vi "Acknowledge Message.vi"(6 "Acknowledge Data":T1, 8 "error in":errorcluster, 9 "Module Action":string, 11 "Module Data In":refnum<class "Rename.lvclass">) -> (0 "error out":errorcluster, 3 "Module Data Out":refnum<class "Rename.lvclass">)   [LabVIEW 2015, in "Generic Module Library.lvlib" / "Template G_Module.lvlib"]
uses:
  Template G_Module.lvlib
  Private Controls/Module Message Cluster Components/Acknowledge Data Cluster.ctl
  Module Class/Rename.lvclass
  Private Controls/Module Message Cluster Components/Ack Payload.ctl
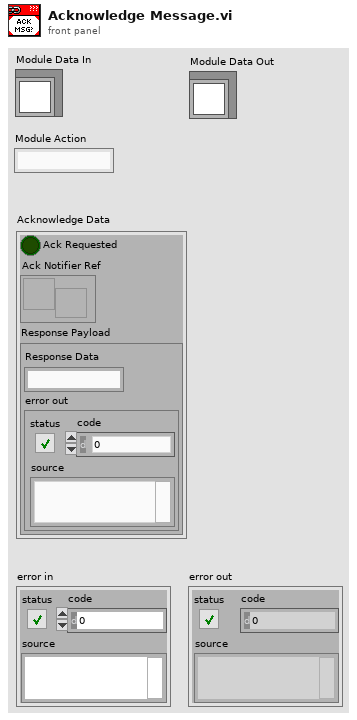
[diagram p1: front panel]
types:
  T1 = typedef "Generic Module Library.lvlib/Template G_Module.lvlib/Acknowledge Data Cluster.ctl" = cluster{"Ack Requested":bool, "Ack Notifier Ref":refnum<notifier>, "Response Payload":T2}
  T2 = typedef "Generic Module Library.lvlib/Template G_Module.lvlib/Ack Payload.ctl" = cluster{"Response Data":string, "error out":errorcluster}
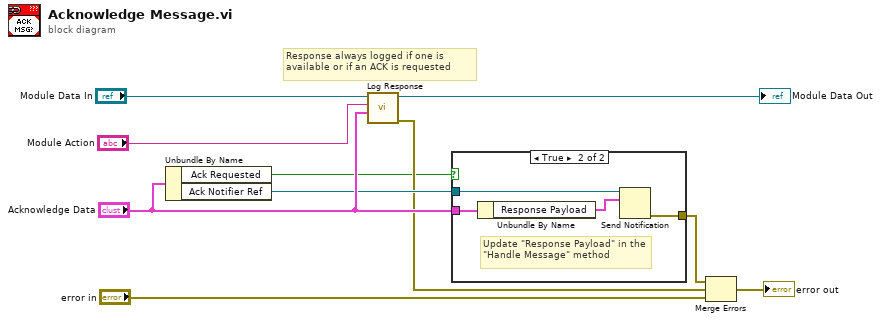
[diagram p0: block diagram]
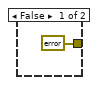
[diagram p2: hidden frame]
diagram:
  # "Response always logged if one is available or if an ACK is requested"
  n1 = Unbundle By Name("Acknowledge Data") -> ("Ack Requested"=w1:bool, "Ack Notifier Ref"=w6:refnum<notifier>)
  n2 = call "Log Response.vi"("Acknowledge Data"="Acknowledge Data", "Module Action"="Module Action", "Module Data In"="Module Data In") -> ("error out"=w3:errorcluster, "Module Data Out"=→"Module Data Out":refnum<class "Rename.lvclass">)  [unwired: 7 in]
  n3 = case shown="True" w1 {
    tunnel: "Acknowledge Data" -> [_ w15]
    tunnel: w6 -> [_ w14]
    tunnel: [errorcluster {"status"=FALSE, "code"=0, "source"=""} ("error out") w12] -> w2
    frame False {
    }
    frame True {
      # "Update \"Response Payload\" in the \"Handle Message\" method"
      n4 = Unbundle By Name(w15) -> ("Response Payload"=w13:T2)
      n5 = Send Notification(notification=w13, notifier=w14) -> (error out=w12:errorcluster)  [unwired: 1 in, 1 out]
    }
  }
  n6 = Merge Errors(w2, w3, "error in") -> (→"error out":errorcluster)
